vi "4155C Config Sampling Measurements FPP.vi"(0 "VISA session":refnum<visa-resource-name>, 1 "Num Points":i16=1 min=1 max=1001, 2 "Vg":dbl min=-100.0 max=100.0 format="%.2f", 3 "Display on/off":bool, 5 "Gate Compliance":dbl format="%.2f", 6 "Sampling mode":u32(slide) scale=0.0..4.0, 9 "Drain Compliance":dbl format="%.2f", 10 "Standby":T1, 11 "error in (no error)":errorcluster, 12 "Timings":T2={"integration time"=0, "Short/Long integration time"=0.00064, "hold time (sec)"=0.0, "delay time (sec)"=0.0, "Step Time (0 disables)"=0.0, "sweep method"=0, "Pulse period"=0.005, "Base voltage"=0.0, "Pulse width"=0.0005} {"Pulse width" min=0.0005 max=0.1 step=0.0001 format="%.4f"; "Base voltage" min=-100.0 max=100.0 format="%^.4e"; "Pulse period" min=0.005 max=1.0 step=0.0001 format="%.4f"; "sweep method" items=["Continuous", "Pulsed"]; "Step Time (0 disables)" format="%.2f"; "delay time (sec)" min=0.0 format="%.4f"; "hold time (sec)" min=0.0 format="%.4f"; "Short/Long integration time" min=0.0 format="%^.0e"; "integration time" scale=0.0..2.0}, 13 "Vd":dbl min=-100.0 max=100.0 format="%.2f", 14 "Sample time":dbl min=0.0 max=100000000000.0 format="%.2f") -> (4 "dup VISA resource name":refnum<visa-resource-name>, 15 "error out":errorcluster)   [LabVIEW 2016]
doc: "This VI configures the primary sweep source (VAR1) for a sweep mode measurement. \n* This VI does not perform error checking on MEASUREMENT MODE or UNIT TYPE of VAR1, therefore it is the application programmer's responsibility to make certain this VI is used in the proper mode."
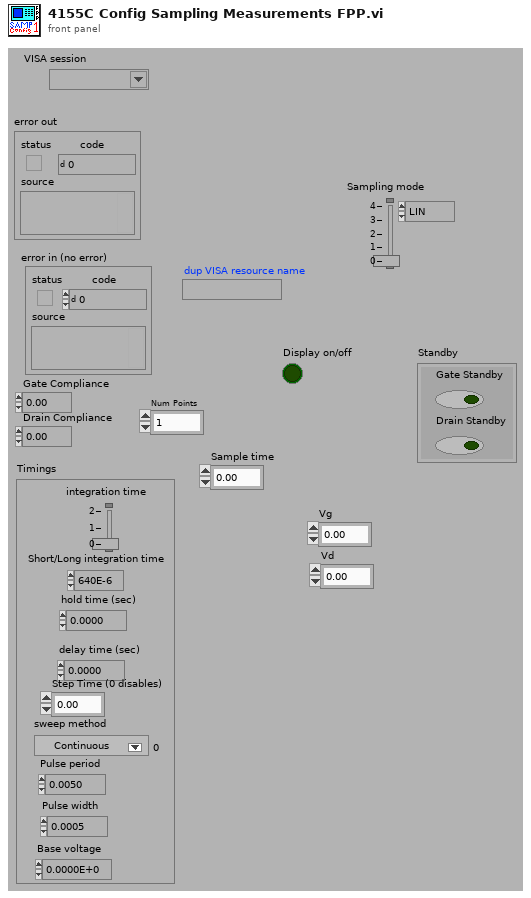
[diagram p1: front panel]
types:
  T1 = cluster{"Gate Standby":bool, "Drain Standby":bool}
  T2 = cluster{"integration time":u32, "Short/Long integration time":dbl, "hold time (sec)":dbl, "delay time (sec)":dbl, "Step Time (0 disables)":dbl, "sweep method":u16, "Pulse period":dbl, "Base voltage":dbl, "Pulse width":dbl}
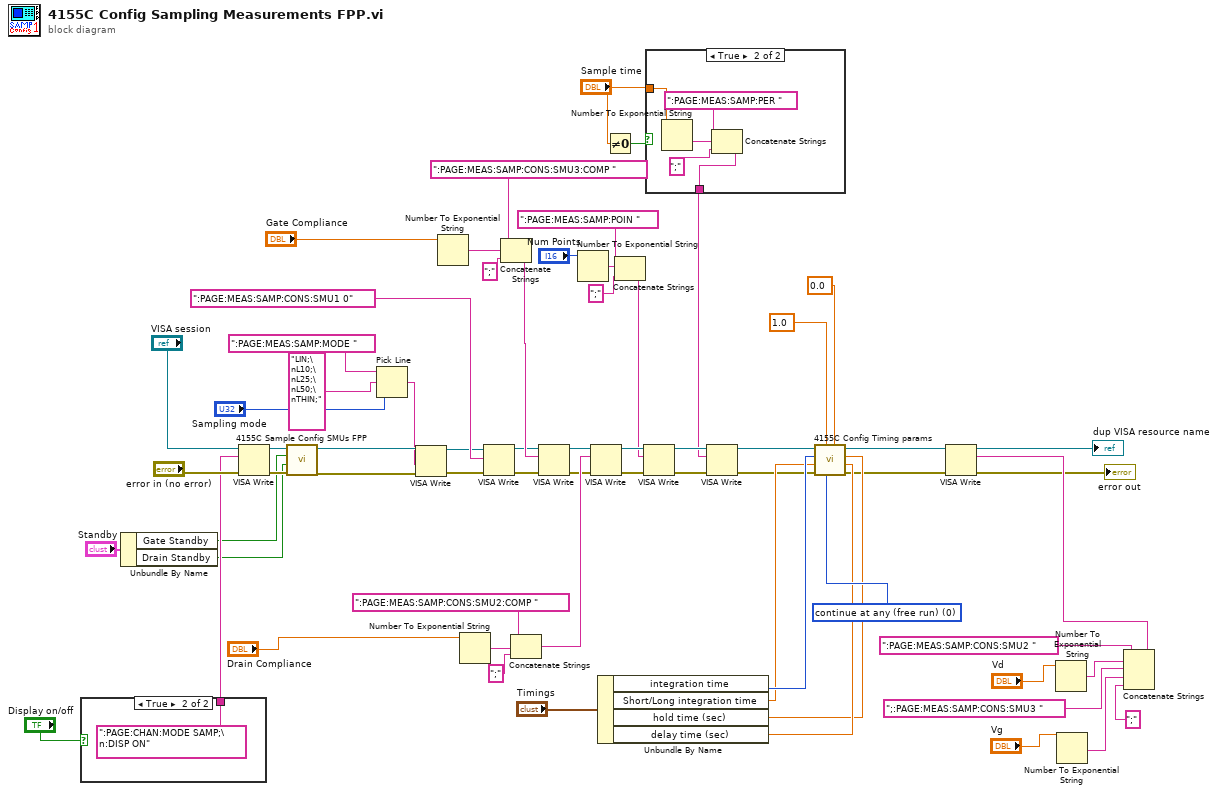
[diagram p0: block diagram]
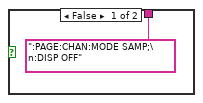
[diagram p2: hidden frame]
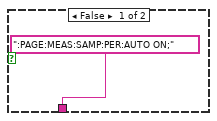
[diagram p3: hidden frame]
diagram:
  w51 = u8 0 items=["continue at any (free run)", "stop at any abnorm", "stop at compliance"] ("stop condition (free run:0)")
  n1 = case shown="True" "Display on/off" {
    tunnel: [":PAGE:CHAN:MODE SAMP;\n:DISP OFF" ("write buffer (\"\")") ":PAGE:CHAN:MODE SAMP;\n:DISP ON" ("write buffer (\"\")")] -> w24
    frame False {
    }
    frame True {
    }
  }
  n2 = Unbundle By Name("Standby") -> ("Gate Standby"=w14:bool, "Drain Standby"=w13:bool)
  n3 = VISA Write(VISA resource name="VISA session", write buffer=w24, error in (no error)="error in (no error)") -> (VISA resource name out=w42:refnum<visa-resource-name>, error out=w41:errorcluster)  [unwired: 1 out]
  n4 = call "4155C Sample Config SMUs FPP.vi"("error in (no error)"=w41, "Drain Standby"=w13, "Gate Standby"=w14, "VISA resource name in"=w42) -> ("error out"=w21:errorcluster, "VISA Resource Name out"=w20:refnum<visa-resource-name>)  [unwired: 6 in]
  n5 = Pick Line(string ("")=":PAGE:MEAS:SAMP:MODE ", multi-line string="LIN;\nL10;\nL25;\nL50;\nTHIN;", line index="Sampling mode") -> (output string=w16:string)
  n6 = VISA Write(VISA resource name=w20, write buffer=w16, error in (no error)=w21) -> (VISA resource name out=w23:refnum<visa-resource-name>, error out=w22:errorcluster)  [unwired: 1 out]
  n7 = Number To Exponential String(number="Gate Compliance") -> (E-format string=w59:string)  [unwired: 3 in]
  n8 = Number To Exponential String(number="Drain Compliance") -> (E-format string=w61:string)  [unwired: 3 in]
  n9 = VISA Write(VISA resource name=w23, write buffer=":PAGE:MEAS:SAMP:CONS:SMU1 0" ("write buffer (\"\")"), error in (no error)=w22) -> (VISA resource name out=w57:refnum<visa-resource-name>, error out=w56:errorcluster)  [unwired: 1 out]
  n10 = Concatenate Strings(":PAGE:MEAS:SAMP:CONS:SMU3:COMP ", w59, ";" ("Substring")) -> (w60:string)
  n11 = Concatenate Strings(":PAGE:MEAS:SAMP:CONS:SMU2:COMP ", w61, ";" ("Substring")) -> (w64:string)
  n12 = VISA Write(VISA resource name=w57, write buffer=w60, error in (no error)=w56) -> (VISA resource name out=w54:refnum<visa-resource-name>, error out=w53:errorcluster)  [unwired: 1 out]
  n13 = Number To Exponential String(number="Num Points") -> (E-format string=w39:string)  [unwired: 3 in]
  n14 = VISA Write(VISA resource name=w54, write buffer=w64, error in (no error)=w53) -> (VISA resource name out=w65:refnum<visa-resource-name>, error out=w66:errorcluster)  [unwired: 1 out]
  n15 = Unbundle By Name("Timings") -> ("integration time"=w48:u32, "Short/Long integration time"=w45:dbl, "hold time (sec)"=w49:dbl, "delay time (sec)"=w50:dbl)
  n16 = Not Equal To 0?(x="Sample time") -> (x != 0?=w31:bool)
  n17 = Concatenate Strings(":PAGE:MEAS:SAMP:POIN " ("write buffer (\"\")"), w39, ";" ("Substring")) -> (w33:string)
  n18 = VISA Write(VISA resource name=w65, write buffer=w33, error in (no error)=w66) -> (VISA resource name out=w30:refnum<visa-resource-name>, error out=w29:errorcluster)  [unwired: 1 out]
  n19 = case shown="True" w31 {
    tunnel: "Sample time" -> [_ w73]
    tunnel: [":PAGE:MEAS:SAMP:PER:AUTO ON;" w70] -> w26
    frame False {
    }
    frame True {
      n20 = Number To Exponential String(number=w73) -> (E-format string=w74:string)  [unwired: 3 in]
      n21 = Concatenate Strings(":PAGE:MEAS:SAMP:PER " ("Substring"), w74, ";" ("Substring")) -> (w70:string)
    }
  }
  n22 = VISA Write(VISA resource name=w30, write buffer=w26, error in (no error)=w29) -> (VISA resource name out=w27:refnum<visa-resource-name>, error out=w28:errorcluster)  [unwired: 1 out]
  n23 = call "4155C Config Timing params.vi"("delay time (sec)"=w50, "hold time (sec)"=w49, "Step Time (0 disables)"=0.0, "stop condition (free run:0)"=w51, "wait time parameter"=1.0, "error in (no error)"=w28, "Short/Long integration time"=w45, "integration time"=w48, "VISA session"=w27) -> ("error out"=w3:errorcluster, "dup VISA resource name"=w4:refnum<visa-resource-name>)  [unwired: 1 in]
  n24 = Number To Exponential String(number="Vd") -> (E-format string=w11:string)  [unwired: 3 in]
  n25 = Number To Exponential String(number="Vg") -> (E-format string=w8:string)  [unwired: 3 in]
  n26 = Concatenate Strings(":PAGE:MEAS:SAMP:CONS:SMU2 " ("write buffer (\"\")"), w11, ";:PAGE:MEAS:SAMP:CONS:SMU3 " ("write buffer (\"\")"), w8, ";" ("Substring")) -> (w7:string)
  n27 = VISA Write(VISA resource name=w4, write buffer=w7, error in (no error)=w3) -> (VISA resource name out=→"dup VISA resource name":refnum<visa-resource-name>, error out=→"error out":errorcluster)  [unwired: 1 out]
